vi "Set Call Registration.vi"(8 "error in (no error)":errorcluster, 10 "Call Registration":T1, 11 "Node in":refnum<class "PyObject.lvclass">) -> (0 "error out":errorcluster, 3 "Node out":refnum<class "PyObject.lvclass">)   [LabVIEW 2020, in "jki_python_bridge.lvlib" / "PyObject.lvclass"]
uses:
  PyObject.lvclass
  Server/Type Definitions/Python Method Call - Event Registration.ctl
  Call/Call.lvclass
  Server/Type Definitions/Public Events - Cluster.ctl
  PyObject.lvclass/PyObject.ctl
  Server/Server.lvclass
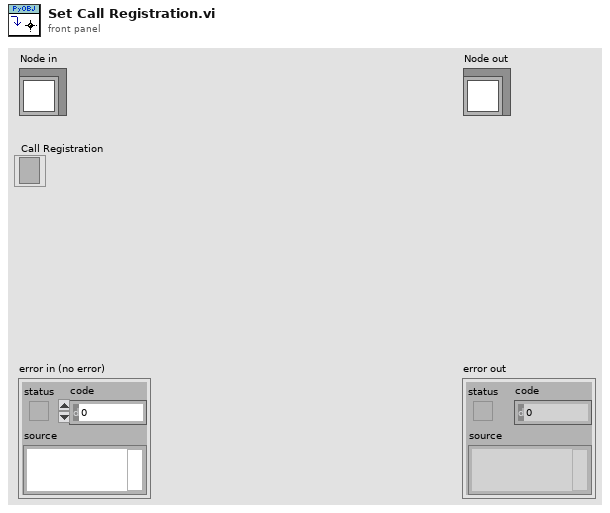
[diagram p1: front panel]
types:
  T1 = typedef "jki_python_bridge.lvlib/Server.lvclass/Python Method Call - Event Registration.ctl" = refnum<event-registration>
  T2 = typedef "jki_python_bridge.lvlib/PyObject.lvclass/Private Data.ctl" = cluster{"Call Registration":T1, "Functions":T3[], "Object Name":string}
  T3 = typedef "JKI_Python_Bridge_for_LV.lvlib/PyObject.lvclass/PyObject Method.ctl" = cluster{"Name":string, "Arguments":string[], "Documentation":string}
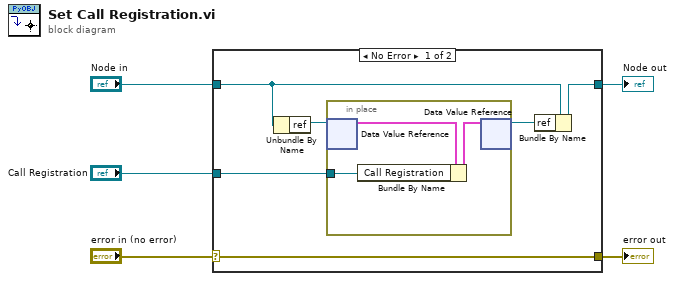
[diagram p0: block diagram]
diagram:
  n1 = case shown="No Error" "error in (no error)" {
    selector: "error in (no error)" -> [w11 w15]
    tunnel: [w11 w15] -> w4
    tunnel: [w8 w16] -> w2
    tunnel: "Node in" -> [w9 w16]
    tunnel: "Call Registration" -> [w6 _]
    frame No Error {
      n2 = Unbundle By Name(w9) -> ("ref"=w10:refnum<data-value>)
      n3 = in-place {
        in-place-border: w6 -> [w12]
        n4 = in-place-dvr #1(w10) -> (w14:T2)  [unwired: 1 out]
        n5 = Bundle By Name(cluster=w14, "Call Registration"=w12) -> (w13:T2)
        n6 = in-place-dvr #1(w13) -> (w7:refnum<data-value>)  [unwired: 1 out]
      }
      n7 = Bundle By Name(cluster=w9, "ref"=w7) -> (w8:refnum<class "PyObject.lvclass">)
    }
    frame Error {
    }
  }
  "error out" <- w4
  "Node out" <- w2
